vi "Log Error.vi"(8 "error in (no error)":errorcluster, 9 "error":errorcluster, 11 "Framework in":refnum<class "Framework.lvclass">) -> (0 "error out":errorcluster, 3 "Framework out":refnum<class "Framework.lvclass">)   [LabVIEW 2017, in "DSF Core.lvlib" / "Framework.lvclass"]
uses:
  Framework.lvclass
  Framework.lvclass/Framework.ctl
  Interface/Logging/Command Data.ctl
  Interface/Logging/Command.ctl
  Interface/Logging/Parameters.ctl
  Interface/Logging/Framework State Parameters.ctl
  Framework States.ctl
  <vilib>/NI/Memory Manager/Classes/Pointer/Pointer.lvclass/Pointer.ctl
  Interface/Interface.lvclass/Interface.ctl
  Interface/Logging/Send Logging Command.vi
  Interface/Send Command.vi
  Interface/Errors.vi
  Interface/Dispatcher/Command Timeout.vi
  <vilib>/NI/Memory Manager/Classes/Pointer/Write.vi
  <vilib>/NI/Memory Manager/Classes/Pointer/Write 1D U8.vi
  <vilib>/NI/Memory Manager/Classes/Pointer/Clear.vi
  Interface/Write RT FIFO.vi
  <vilib>/NI/Memory Manager/Classes/Pointer/Write (No Check).vi
  <vilib>/NI/Memory Manager/Classes/Pointer/Write (No Check) 1D U8.vi
  <vilib>/NI/Memory Manager/Classes/Pointer/Check Move.vi
  <vilib>/NI/Memory Manager/Classes/Pointer/Check Null Pointer.vi
  <vilib>/NI/Memory Manager/Classes/Pointer/Clear (No Check).vi
  <vilib>/NI/Memory Manager/Classes/Pointer/Check Length.vi
  <vilib>/NI/Memory Manager/Classes/Pointer/Check Count.vi
  <vilib>/NI/Memory Manager/Classes/Pointer/Check Bounds (Power of 2).vi
  <vilib>/NI/Memory Manager/Classes/Pointer/Errors.vi
  <vilib>/NI/Memory Manager/Classes/Pointer/Null Pointer.vi
  <vilib>/NI/Memory Manager/Classes/Pointer/Is Null.vi
  <vilib>/NI/Memory Manager/Classes/Pointer/Get Size.vi
  <vilib>/NI/Memory Manager/Classes/Pointer/Check Bounds (Pointer).vi
  <vilib>/NI/Memory Manager/Classes/Pointer/Out of Bounds.vi
  <vilib>/NI/Memory Manager/Classes/Pointer/Check Bounds.vi
  <vilib>/NI/Memory Manager/Classes/Pointer/Create Error.vi
  <vilib>/NI/Memory Manager/Classes/Pointer/Write Pointer Size to Error.vi
  <vilib>/NI/Memory Manager/Classes/Pointer/Check Bounds (Buffer).vi
  <vilib>/NI/Memory Manager/Constants/Constants.vi
  <vilib>/NI/Memory Manager/Constants/Library Name.vi
  <vilib>/NI/Memory Manager/Classes/Pointer/Pointer Error Info.vi
  <vilib>/NI/Memory Manager/Constants/Pointer Class Name.vi
  <vilib>/NI/Memory Manager/Classes/Pointer/Buffer Underflow.vi
  Pointers/Error/Error Pointer.lvclass
  C:/Program Files (x86)/National Instruments/LabVIEW 2017/vi.lib/NI/Memory Manager/Classes/Pointer/Pointer.lvclass
  Interface/Logging/Logging Interface.lvclass
  C:/Git/DSF/Core/Classes/Interface/Interface.lvclass
  Interface/New Interface Error.vi
  VIs/VI Name.vi
  <vilib>/NI/Memory Manager/VIs/Write String to Source.vi
  <vilib>/NI/Memory Manager/VIs/Write Numeric to Source.vi
  <vilib>/NI/Memory Manager/VIs/Write Numeric Scalar to Source (Base10 U64).vi
  <vilib>/NI/Memory Manager/VIs/Set Error Source.vi
  <vilib>/NI/Memory Manager/VIs/Set Error Code.vi
  <vilib>/NI/Memory Manager/VIs/Set Error Status.vi
  <vilib>/NI/Memory Manager/VIs/New Error Cluster.vi
  <vilib>/NI/Memory Manager/VIs/New Error Cluster (512B).vi
  <vilib>/NI/Memory Manager/Classes/Pointer/Pointer.lvclass
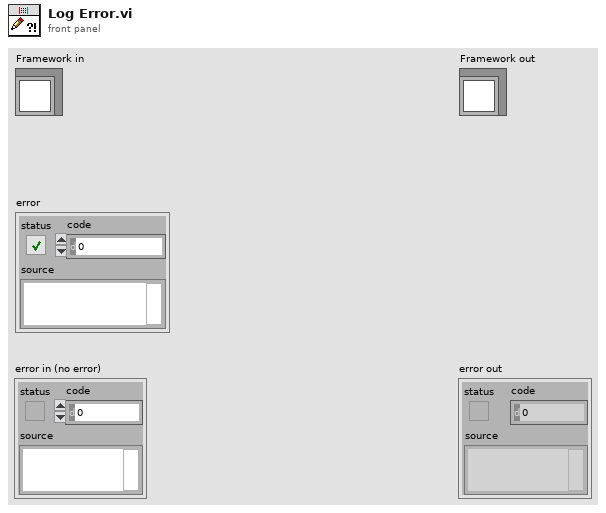
[diagram p1: front panel]
types:
  T1 = typedef "DSF Core.lvlib/Logging Interface.lvclass/Parameters.ctl" = cluster{"arg1":u64, "arg2":u64}
  T2 = typedef "DSF Core.lvlib/Logging Interface.lvclass/Framework State Parameters.ctl" = cluster{"state":T3, "unused":u8, "unused 2":u16, "unused 3":u32, "error pointer":u64}
  T3 = typedef "DSF Core.lvlib/Framework.lvclass/Framework States.ctl" = enum8{"Uninitialized", "Initialized", "Running", "Error", "Shut Down"}
  T4 = typedef "DSF Core.lvlib/Logging Interface.lvclass/Command.ctl" = enum8{"Idle", "Start", "Log Framework State", "Log Plugin State", "Log Dispatcher State", "Shutdown"}
  T5 = typedef "DSF Core.lvlib/Logging Interface.lvclass/Command Data.ctl" = cluster{"Command":T4, "Parameters":T1}
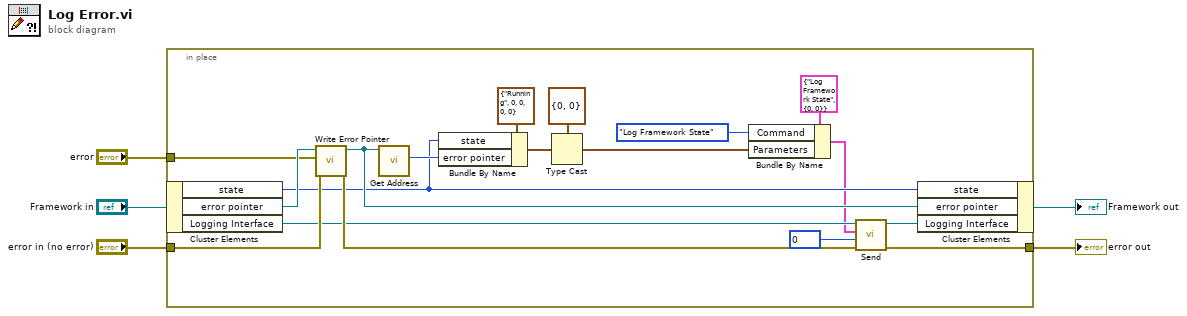
[diagram p0: block diagram]
diagram:
  n1 = in-place {
    in-place-border: [w18] -> w5
    in-place-border: "error in (no error)" -> [w22]
    in-place-border: "error" -> [w8]
    n2 = in-place-cluster #1("Framework in") -> ("state"=w7:T3, "error pointer"=w11:refnum<class "Error Pointer.lvclass">, "Logging Interface"=w21:refnum<class "Logging Interface.lvclass">)
    n3 = call "Write Error Pointer.vi"("error in (no error)"=w22, "error"=w8, "Error Pointer in"=w11) -> ("error out"=w23:errorcluster, "Error Pointer in"=w9:refnum<class "Error Pointer.lvclass">)  [unwired: 7 in]
    n4 = call <vilib>:"Get Address.vi"("Pointer in"=w9) -> ("address"=w10:u64)  [unwired: 9 in, 1 out]
    n5 = Bundle By Name(cluster=T2 {"state"=enum."Running", "unused"=0, "unused 2"=0, "unused 3"=0, "error pointer"=0} ("Parameters"), "state"=w7, "error pointer"=w10) -> (w15:T2)
    n6 = Type Cast(type=T1 {"arg1"=0, "arg2"=0} ("Parameters"), x=w15) -> (*(type *) &x=w13:T1)
    n7 = Bundle By Name(cluster=T5 {"Command"=enum."Log Framework State", "Parameters"={"arg1"=0, "arg2"=0}} ("command"), "Command"=Command."Log Framework State", "Parameters"=w13) -> (w6:T5)
    n8 = call-poly "Send.vi"("error in (no error)"=w23, "timeout in ms (0)"=0, "command"=w6, "Logging Interface in"=w21) -> ("error out"=w18:errorcluster, "Logging Interface out"=w17:refnum<class "Logging Interface.lvclass">)  [unwired: 6 in]
    n9 = in-place-cluster #1("state"=w7, "error pointer"=w9, "Logging Interface"=w17) -> (→"Framework out":refnum<class "Framework.lvclass">)
  }
  "error out" <- w5
